vi "Read Sensors V.3.0.vi"(1 "Left Dart Motor":T1={"DeviceStatus"={"status"=FALSE, "code"=0, "source"=""}, "Type"=enum."PWM", "PWM"={"PWM Channel"=enum."Invalid", "DeadBand"={"Name"="", "maxPositivePwm"=0, "minPositivePwm"=0, "centerPwm"=0, "maxNegativePwm"=0, "minNegativePwm"=0, "angularRange"=0}}, "CAN"={"Device Number"=0, "SetOutput VI Ref"=variant(enum8{"Percent VBus", "Current", "Speed", "Position", "Voltage"} enum."Percent VBus"), "GetOutput VI Ref"=variant(refnum<k1> refnum), "Enable VI Ref"=variant(dbl 12.0), "Disable VI Ref"=variant(enum8{"Percent VBus", "Speed", "Position", "Slave", "Unchanged / Invalid", "Voltage Compensation", "Current", "Motion Profile"} enum."Percent VBus"), "Data"=variant}, "Invert"=FALSE, "DIO PWM"={"PWM \"Enable\" Channel"=enum."Invalid", "DIOChannel"=enum."Invalid", "PWM Rate"=0.0}}, 2 "Right Dart Motor":T1={"DeviceStatus"={"status"=FALSE, "code"=0, "source"=""}, "Type"=enum."PWM", "PWM"={"PWM Channel"=enum."Invalid", "DeadBand"={"Name"="", "maxPositivePwm"=0, "minPositivePwm"=0, "centerPwm"=0, "maxNegativePwm"=0, "minNegativePwm"=0, "angularRange"=0}}, "CAN"={"Device Number"=0, "SetOutput VI Ref"=variant(enum8{"Percent VBus", "Current", "Speed", "Position", "Voltage"} enum."Percent VBus"), "GetOutput VI Ref"=variant(refnum<k1> refnum), "Enable VI Ref"=variant(dbl 12.0), "Disable VI Ref"=variant(enum8{"Percent VBus", "Speed", "Position", "Slave", "Unchanged / Invalid", "Voltage Compensation", "Current", "Motion Profile"} enum."Percent VBus"), "Data"=variant}, "Invert"=FALSE, "DIO PWM"={"PWM \"Enable\" Channel"=enum."Invalid", "DIOChannel"=enum."Invalid", "PWM Rate"=0.0}}, 3 "Right Collector Intake Motor":T1={"DeviceStatus"={"status"=FALSE, "code"=0, "source"=""}, "Type"=enum."PWM", "PWM"={"PWM Channel"=enum."Invalid", "DeadBand"={"Name"="", "maxPositivePwm"=0, "minPositivePwm"=0, "centerPwm"=0, "maxNegativePwm"=0, "minNegativePwm"=0, "angularRange"=0}}, "CAN"={"Device Number"=0, "SetOutput VI Ref"=variant(enum8{"Percent VBus", "Current", "Speed", "Position", "Voltage"} enum."Percent VBus"), "GetOutput VI Ref"=variant(refnum<k1> refnum), "Enable VI Ref"=variant(dbl 12.0), "Disable VI Ref"=variant(enum8{"Percent VBus", "Speed", "Position", "Slave", "Unchanged / Invalid", "Voltage Compensation", "Current", "Motion Profile"} enum."Percent VBus"), "Data"=variant}, "Invert"=FALSE, "DIO PWM"={"PWM \"Enable\" Channel"=enum."Invalid", "DIOChannel"=enum."Invalid", "PWM Rate"=0.0}}, 4 "Right Pot.":T6, 5 "Left Collector Intake Motor":T1={"DeviceStatus"={"status"=FALSE, "code"=0, "source"=""}, "Type"=enum."PWM", "PWM"={"PWM Channel"=enum."Invalid", "DeadBand"={"Name"="", "maxPositivePwm"=0, "minPositivePwm"=0, "centerPwm"=0, "maxNegativePwm"=0, "minNegativePwm"=0, "angularRange"=0}}, "CAN"={"Device Number"=0, "SetOutput VI Ref"=variant(enum8{"Percent VBus", "Current", "Speed", "Position", "Voltage"} enum."Percent VBus"), "GetOutput VI Ref"=variant(refnum<k1> refnum), "Enable VI Ref"=variant(dbl 12.0), "Disable VI Ref"=variant(enum8{"Percent VBus", "Speed", "Position", "Slave", "Unchanged / Invalid", "Voltage Compensation", "Current", "Motion Profile"} enum."Percent VBus"), "Data"=variant}, "Invert"=FALSE, "DIO PWM"={"PWM \"Enable\" Channel"=enum."Invalid", "DIOChannel"=enum."Invalid", "PWM Rate"=0.0}}, 6 "Left Pot.":T6) -> ()   [LabVIEW 2017]
uses:
  <vilib>/Rock Robotics/WPI/Potentiometer/WPI_PotentiometerDevRef.ctl
  <vilib>/Rock Robotics/SystemInterfaces/AI/FPGA_AIChannel.ctl
  <vilib>/Rock Robotics/WPI/MotorControl/WPI_MotorControlDeviceRef.ctl
  <vilib>/Rock Robotics/WPI/MotorControl/WPI_MotorControlType.ctl
  <vilib>/Rock Robotics/SystemInterfaces/DIO/FPGA_DIOPWMChannel.ctl
  <vilib>/Rock Robotics/WPI/PWM/WPI_PWMDeadband.ctl
  <vilib>/Rock Robotics/SystemInterfaces/DIO/FPGA_DIOChannel.ctl
  Robot Global Data V.3.0.vi
  Public/Documents/Cross The Road Electronics/Phoenix-LabVIEW/Motor Controller/Get/CTRE_Phoenix_MotorController_GetOutputCurrent_Enhanced.vi
  Public/Documents/Cross The Road Electronics/Phoenix-LabVIEW/Motor Controller/Get/CTRE_Phoenix_MotorController_GetQuadratureData.vi
  <vilib>/Rock Robotics/WPI/Utilities/WPI_GetSetVariantRefNum.vi
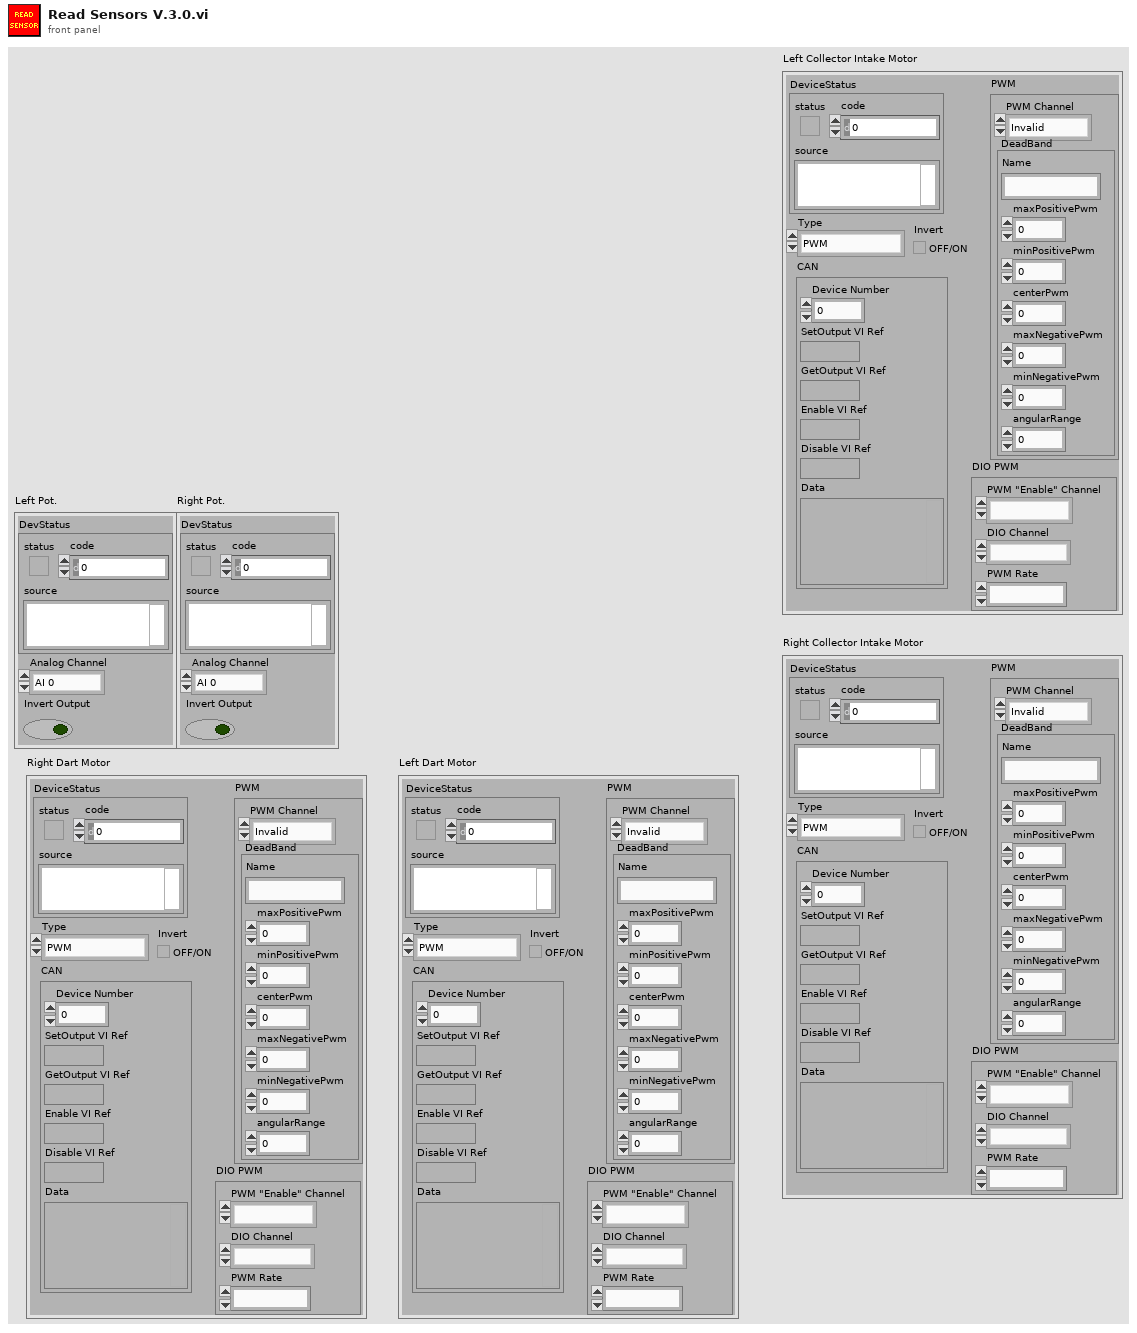
[diagram p1: front panel]
types:
  T1 = typedef "WPI_MotorControlDeviceRef.ctl" = cluster{"DeviceStatus":errorcluster, "Type":T2, "PWM":cluster{"PWM Channel":T3, "DeadBand":T4}, "CAN":cluster{"Device Number":u8, "SetOutput VI Ref":variant, "GetOutput VI Ref":variant, "Enable VI Ref":variant, "Disable VI Ref":variant, "Data":variant}, "Invert":bool, "DIO PWM":cluster{"PWM \"Enable\" Channel":T3, "DIOChannel":T5, "PWM Rate":dbl}}
  T2 = typedef "WPI_MotorControlType.ctl" = enum16{"PWM", "CAN", "DIO PWM"}
  T3 = typedef "FPGA_DIOPWMChannel.ctl" = enum8{"PWM 0", "PWM 1", "PWM 2", "PWM 3", "PWM 4", "PWM 5", "PWM 6", "PWM 7", "PWM 8", "PWM 9", "PWM MXP 0", "PWM MXP 1", "PWM MXP 2", "PWM MXP 3", "PWM MXP 4", "PWM MXP 5", "PWM MXP 6", "PWM MXP 7", "PWM MXP 8", "PWM MXP 9", "Invalid"}
  T4 = typedef "WPI_PWMDeadband.ctl" = cluster{"Name":string, "maxPositivePwm":i32, "minPositivePwm":i32, "centerPwm":i32, "maxNegativePwm":i32, "minNegativePwm":i32, "angularRange":u16}
  T5 = typedef "FPGA_DIOChannel.ctl" = enum8{"DIO 0", "DIO 1", "DIO 2", "DIO 3", "DIO 4", "DIO 5", "DIO 6", "DIO 7", "DIO 8", "DIO 9", "DIO MXP 0", "DIO MXP 1", "DIO MXP 2", "DIO MXP 3", "DIO MXP 4", "DIO MXP 5", "DIO MXP 6", "DIO MXP 7", "DIO MXP 8", "DIO MXP 9", "DIO MXP 10", "DIO MXP 11", "DIO MXP 12", "DIO MXP 13", "DIO MXP 14", "DIO MXP 15", "SPI Port CS1", "SPI Port CS2", "SPI Port CS3", "SPI Port MISO", "SPI Port MOSI", "Invalid"}
  T6 = typedef "WPI_PotentiometerDevRef.ctl" = cluster{"DevStatus":errorcluster, "Analog Channel":T7, "Invert Output":bool}
  T7 = typedef "FPGA_AIChannel.ctl" = enum8{"AI 0", "AI 1", "AI 2", "AI 3", "AI MXP 0", "AI MXP 1", "AI MXP 2", "AI MXP 3", "Invalid"}
  T8 = cluster{"Pot. Voltage":dbl[], "Corresponding Inches":dbl[]}
  T9 = typedef "WPI_RobotDriveDevRef.ctl" = cluster{"DevStatus":errorcluster, "Motors[]":T1[], "Square Inputs":bool, "Max Output":dbl}
  T10 = typedef "WPI_GyroDevRef.ctl" = cluster{"DevStatus":errorcluster, "Analog Channel":T7, "Gain (VoltsPerDegree/Second)":dbl, "Gyro Type":enum16{"Analog", "XRS450"}, "Handle":i32, "SPI Bus":T11, "Device Found":bool, "Sample Rate":dbl, "Calibrate On Open":bool, "Offset":dbl}
  T11 = typedef "spi_bus.ctl" = enum16{"SPI On-Board, CS0", "SPI On-Board, CS1", "SPI On-Board, CS2", "SPI On-Board, CS3", "SPI MXP", "Invalid"}
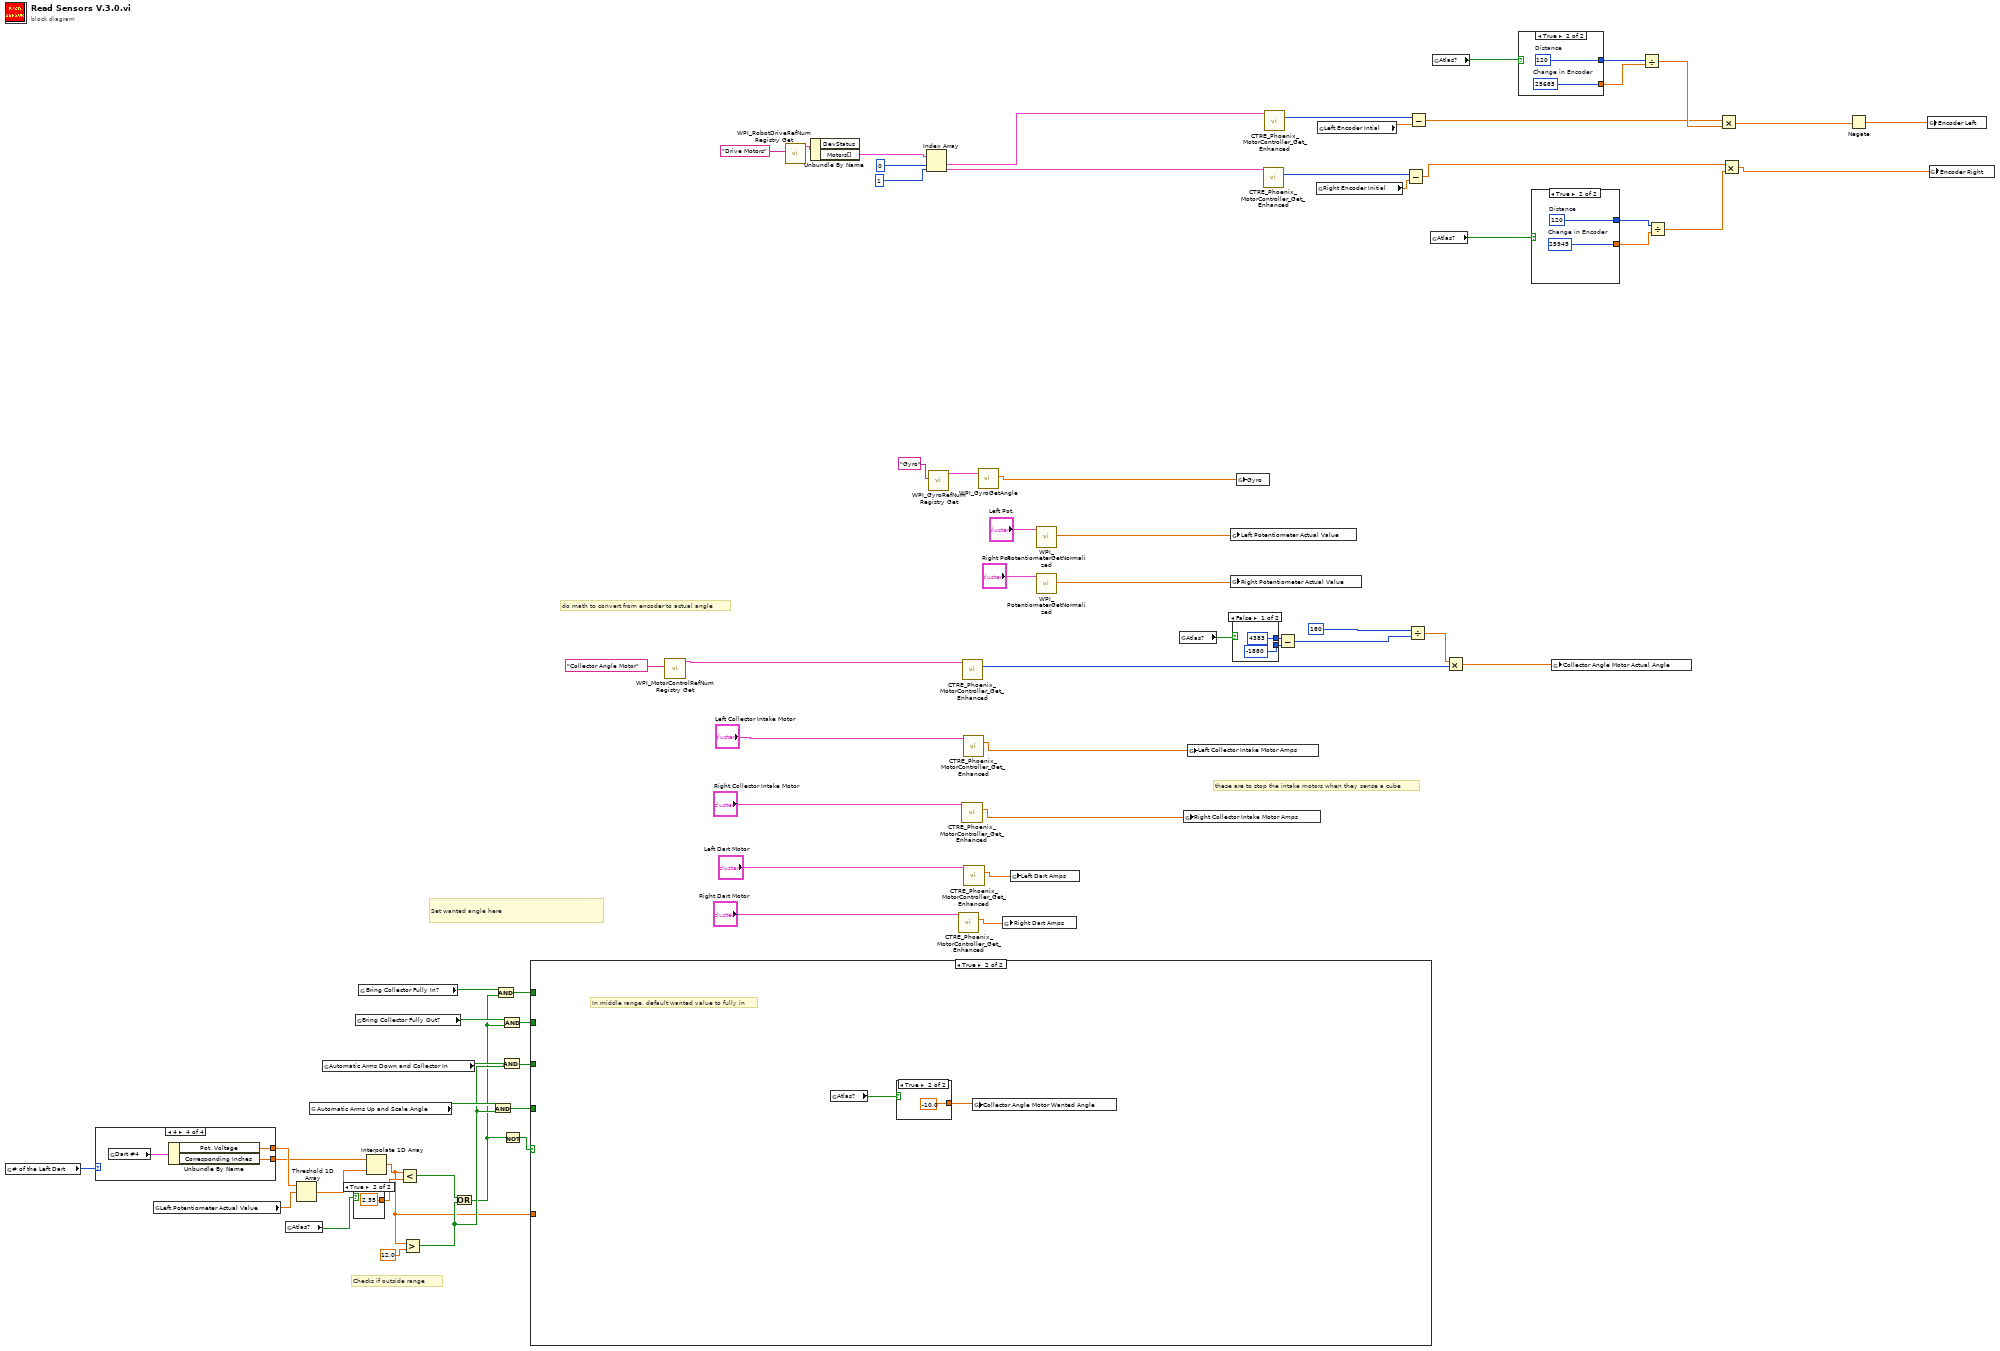
[diagram p0: block diagram]
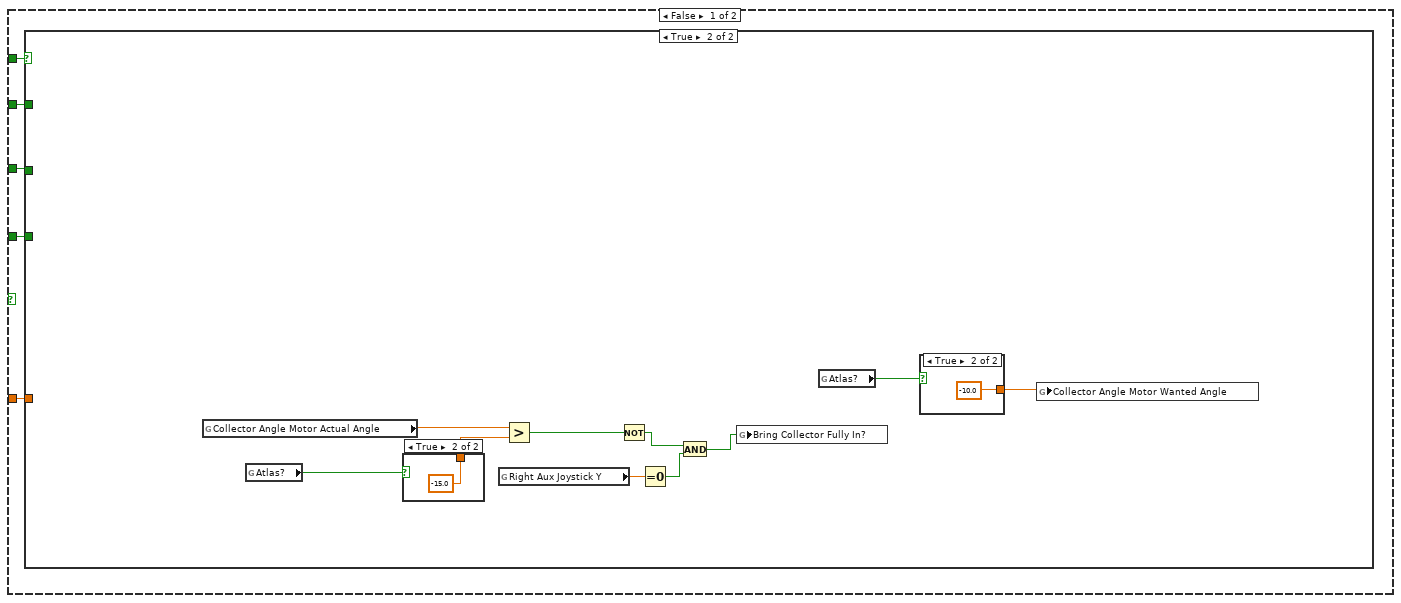
[diagram p2: hidden frame]
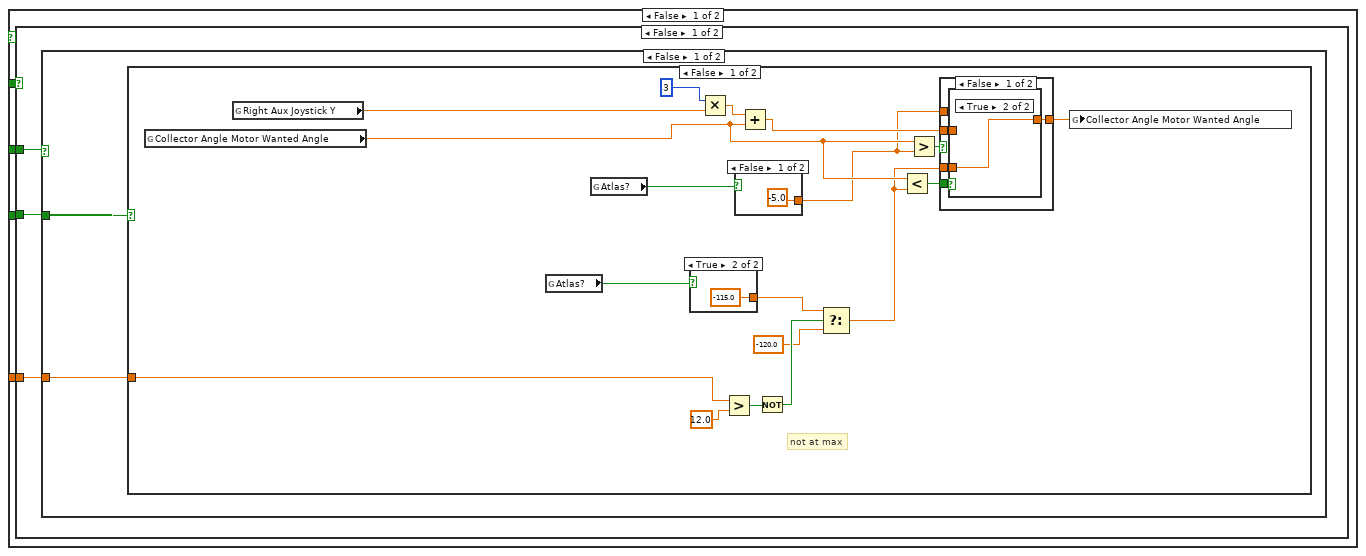
[diagram p3: hidden frame]
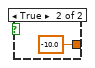
[diagram p4: hidden frame]
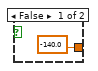
[diagram p5: hidden frame]
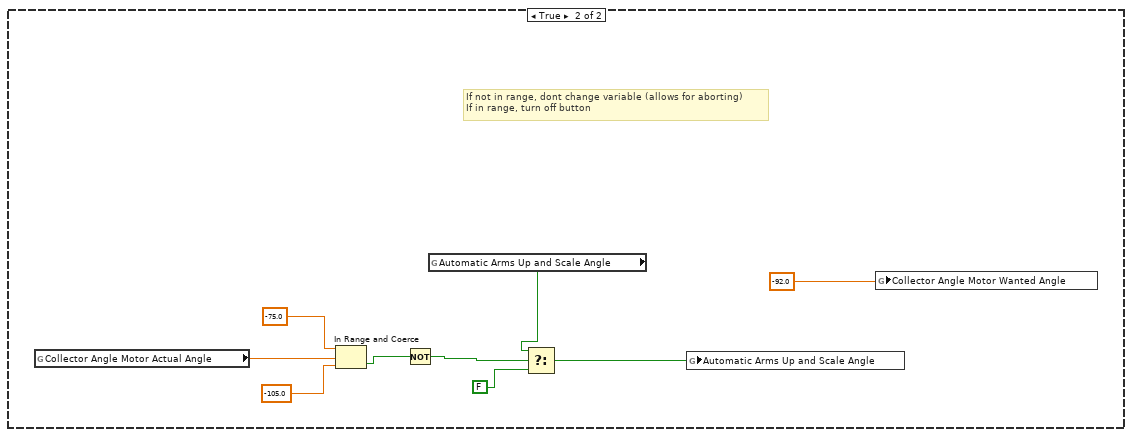
[diagram p8: hidden frame]
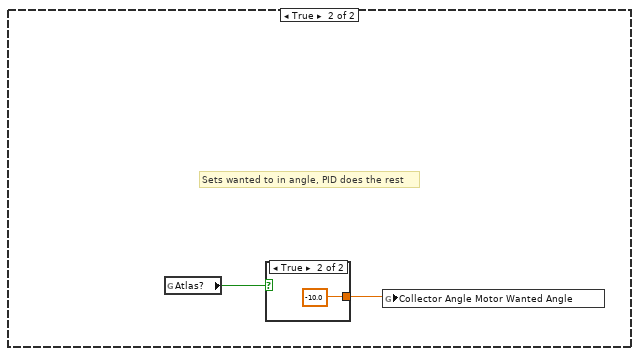
[diagram p9: hidden frame]
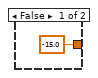
[diagram p10: hidden frame]
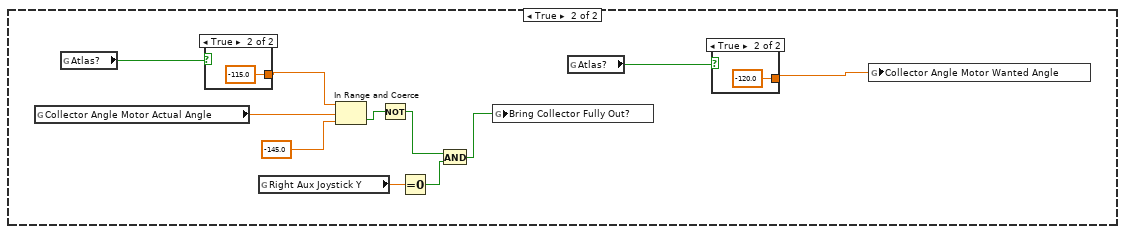
[diagram p11: hidden frame]
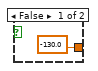
[diagram p12: hidden frame]
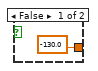
[diagram p13: hidden frame]
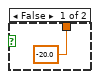
[diagram p14: hidden frame]
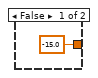
[diagram p15: hidden frame]
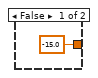
[diagram p16: hidden frame]
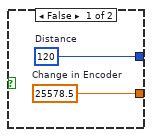
[diagram p17: hidden frame]
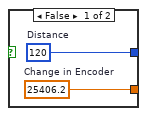
[diagram p18: hidden frame]
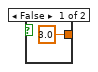
[diagram p19: hidden frame]
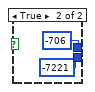
[diagram p20: hidden frame]
diagram:
  # "Checks if outside range"
  # "Set wanted angle here"
  # "these are to stop the intake motors when they sense a cube"
  # "do math to convert from encoder to actual angle"
  n1 = global read "Robot Global Data V.3.0.vi" "# of the Left Dart"() -> (w29:i32)
  n2 = case shown="4" w29 {
    tunnel: [w72 w75 w78 w81] -> w31
    tunnel: [w71 w74 w77 w80] -> w30
    frame 1, Default {
      n3 = global read "Robot Global Data V.3.0.vi" "Dart #1"() -> (w73:T8)
      n4 = Unbundle By Name(w73) -> ("Pot. Voltage"=w72:dbl[], "Corresponding Inches"=w71:dbl[])
    }
    frame 2 {
      n5 = global read "Robot Global Data V.3.0.vi" "Dart #2"() -> (w76:T8)
      n6 = Unbundle By Name(w76) -> ("Pot. Voltage"=w75:dbl[], "Corresponding Inches"=w74:dbl[])
    }
    frame 3 {
      n7 = global read "Robot Global Data V.3.0.vi" "Dart #3"() -> (w79:T8)
      n8 = Unbundle By Name(w79) -> ("Pot. Voltage"=w78:dbl[], "Corresponding Inches"=w77:dbl[])
    }
    frame 4 {
      n9 = global read "Robot Global Data V.3.0.vi" "Dart #4"() -> (w82:T8)
      n10 = Unbundle By Name(w82) -> ("Pot. Voltage"=w81:dbl[], "Corresponding Inches"=w80:dbl[])
    }
  }
  n11 = global read "Robot Global Data V.3.0.vi" "Left Potentiometer Actual Value"() -> (w32:dbl)
  n12 = global read "Robot Global Data V.3.0.vi" "Atlas?"() -> (w14:bool)
  n13 = Threshold 1D Array(2:w32, 3:w31) -> (0:w33:dbl)  [unwired: 1 in]
  n14 = global read "Robot Global Data V.3.0.vi" "Automatic Arms Up and Scale Angle"() -> (w16:bool)
  n15 = global read "Robot Global Data V.3.0.vi" "Automatic Arms Down and Collector In"() -> (w8:bool)
  n16 = case shown="True" w14 {
    tunnel: [3.0 ("y") 2.35 ("y")] -> w28
    frame False {
    }
    frame True {
    }
  }
  n17 = global read "Robot Global Data V.3.0.vi" "Bring Collector Fully Out?"() -> (w24:bool)
  n18 = global read "Robot Global Data V.3.0.vi" "Bring Collector Fully In?"() -> (w25:bool)
  n19 = Interpolate 1D Array(1:w33, 2:w30) -> (0:w3:dbl)
  n20 = Less?(x=w3, y=w28) -> (x < y?=w26:bool)
  n21 = Greater?(x=w3, y=12.0) -> (0:w6:bool)
  n22 = Or(x=w26, y=w6) -> (x .or. y?=w1:bool)
  n23 = And(x=w16, y=w6) -> (x .and. y?=w11:bool)
  n24 = And(x=w25, y=w1) -> (x .and. y?=w13:bool)
  n25 = And(x=w8, y=w6) -> (x .and. y?=w7:bool)
  n26 = And(x=w24, y=w1) -> (x .and. y?=w12:bool)
  n27 = Not(x=w1) -> (.not. x?=w2:bool)
  n28 = case shown="True" w2 {
    tunnel: w13 -> [w89 _]
    tunnel: w12 -> [w88 _]
    tunnel: w11 -> [w87 _]
    tunnel: w7 -> [w86 _]
    tunnel: w3 -> [w85 _]
    frame False {
      n29 = case shown="True" w89 {
        tunnel: w88 -> [w93 _]
        tunnel: w86 -> [w92 _]
        tunnel: w87 -> [w91 _]
        tunnel: w85 -> [w90 _]
        frame False {
          n30 = case shown="False" w93 {
            tunnel: w92 -> [w96 _]
            tunnel: w91 -> [w95 _]
            tunnel: w90 -> [w94 _]
            frame False {
              n31 = case shown="False" w96 {
                tunnel: w95 -> [w98 _]
                tunnel: w94 -> [w97 _]
                frame False {
                  n32 = case shown="False" w98 {
                    tunnel: w97 -> [w101 _]
                    frame False {
                      # "not at max"
                      n33 = global read "Robot Global Data V.3.0.vi" "Collector Angle Motor Wanted Angle"() -> (w110:dbl)
                      n34 = global read "Robot Global Data V.3.0.vi" "Right Aux Joystick Y"() -> (w116:dbl)
                      n35 = global read "Robot Global Data V.3.0.vi" "Atlas?"() -> (w102:bool)
                      n36 = global read "Robot Global Data V.3.0.vi" "Atlas?"() -> (w100:bool)
                      n37 = case shown="True" w102 {
                        tunnel: [-140.0 ("t") -115.0 ("t")] -> w105
                        frame False {
                        }
                        frame True {
                        }
                      }
                      n38 = Multiply(x=3, y=w116) -> (x*y=w115:dbl)
                      n39 = Greater?(x=w101, y=12.0) -> (0:w107:bool)
                      n40 = case shown="False" w100 {
                        tunnel: [-5.0 ("t") -10.0 ("t")] -> w99
                        frame False {
                        }
                        frame True {
                        }
                      }
                      n41 = Add(x=w115, y=w110) -> (x+y=w113:dbl)
                      n42 = Not(x=w107) -> (.not. x?=w106:bool)
                      n43 = Select(t=w105, s=w106, f=-120.0) -> (s? t:f=w103:dbl)
                      n44 = Less?(x=w110, y=w103) -> (x < y?=w109:bool)
                      n45 = Greater?(x=w110, y=w99) -> (0:w112:bool)
                      n46 = case shown="False" w112 {
                        tunnel: w99 -> [_ w127]
                        tunnel: w113 -> [w121 _]
                        tunnel: [w123 w127] -> w111
                        tunnel: w109 -> [w124 _]
                        tunnel: w103 -> [w122 _]
                        frame False {
                          n47 = case shown="True" w124 {
                            tunnel: [w125 w126] -> w123
                            tunnel: w122 -> [_ w126]
                            tunnel: w121 -> [w125 _]
                            frame False {
                            }
                            frame True {
                            }
                          }
                        }
                        frame True {
                        }
                      }
                      n48 = global write "Robot Global Data V.3.0.vi" "Collector Angle Motor Wanted Angle"(w111) -> ()
                    }
                    frame True {
                      # "If not in range, dont change variable (allows for aborting)\nIf in range, turn off button"
                      n49 = global read "Robot Global Data V.3.0.vi" "Collector Angle Motor Actual Angle"() -> (w134:dbl)
                      n50 = In Range and Coerce(upper limit=-75.0, x=w134, lower limit=-105.0) -> (In Range?=w135:bool)  [unwired: 1 out]
                      n51 = Not(x=w135) -> (.not. x?=w131:bool)
                      n52 = global read "Robot Global Data V.3.0.vi" "Automatic Arms Up and Scale Angle"() -> (w129:bool)
                      n53 = Select(t=w129, s=w131, f=FALSE) -> (s? t:f=w130:bool)
                      n54 = global write "Robot Global Data V.3.0.vi" "Automatic Arms Up and Scale Angle"(w130) -> ()
                      n55 = global write "Robot Global Data V.3.0.vi" "Collector Angle Motor Wanted Angle"(-92.0) -> ()
                    }
                  }
                }
                frame True {
                  # "Sets wanted to in angle, PID does the rest"
                  n56 = global read "Robot Global Data V.3.0.vi" "Atlas?"() -> (w137:bool)
                  n57 = case shown="True" w137 {
                    tunnel: [-15.0 -10.0] -> w138
                    frame False {
                    }
                    frame True {
                    }
                  }
                  n58 = global write "Robot Global Data V.3.0.vi" "Collector Angle Motor Wanted Angle"(w138) -> ()
                }
              }
            }
            frame True {
              n59 = global read "Robot Global Data V.3.0.vi" "Collector Angle Motor Actual Angle"() -> (w150:dbl)
              n60 = global read "Robot Global Data V.3.0.vi" "Atlas?"() -> (w142:bool)
              n61 = case shown="True" w142 {
                tunnel: [-130.0 ("t") -115.0 ("t")] -> w141
                frame False {
                }
                frame True {
                }
              }
              n62 = global read "Robot Global Data V.3.0.vi" "Right Aux Joystick Y"() -> (w148:dbl)
              n63 = In Range and Coerce(upper limit=w141, x=w150, lower limit=-145.0) -> (In Range?=w151:bool)  [unwired: 1 out]
              n64 = Not(x=w151) -> (.not. x?=w146:bool)
              n65 = Equal To 0?(x=w148) -> (x = 0?=w147:bool)
              n66 = And(x=w146, y=w147) -> (x .and. y?=w145:bool)
              n67 = global write "Robot Global Data V.3.0.vi" "Bring Collector Fully Out?"(w145) -> ()
              n68 = global read "Robot Global Data V.3.0.vi" "Atlas?"() -> (w144:bool)
              n69 = case shown="True" w144 {
                tunnel: [-130.0 ("t") -120.0 ("t")] -> w143
                frame False {
                }
                frame True {
                }
              }
              n70 = global write "Robot Global Data V.3.0.vi" "Collector Angle Motor Wanted Angle"(w143) -> ()
            }
          }
        }
        frame True {
          n71 = global read "Robot Global Data V.3.0.vi" "Collector Angle Motor Actual Angle"() -> (w163:dbl)
          n72 = global read "Robot Global Data V.3.0.vi" "Atlas?"() -> (w161:bool)
          n73 = case shown="True" w161 {
            tunnel: [-20.0 -15.0] -> w162
            frame False {
            }
            frame True {
            }
          }
          n74 = global read "Robot Global Data V.3.0.vi" "Right Aux Joystick Y"() -> (w159:dbl)
          n75 = Greater?(x=w163, y=w162) -> (0:w164:bool)
          n76 = Not(x=w164) -> (.not. x?=w157:bool)
          n77 = Equal To 0?(x=w159) -> (x = 0?=w158:bool)
          n78 = And(x=w157, y=w158) -> (x .and. y?=w156:bool)
          n79 = global write "Robot Global Data V.3.0.vi" "Bring Collector Fully In?"(w156) -> ()
          n80 = global read "Robot Global Data V.3.0.vi" "Atlas?"() -> (w160:bool)
          n81 = case shown="True" w160 {
            tunnel: [-15.0 -10.0] -> w165
            frame False {
            }
            frame True {
            }
          }
          n82 = global write "Robot Global Data V.3.0.vi" "Collector Angle Motor Wanted Angle"(w165) -> ()
        }
      }
    }
    frame True {
      # "In middle range, default wanted value to fully in"
      n83 = global read "Robot Global Data V.3.0.vi" "Atlas?"() -> (w170:bool)
      n84 = case shown="True" w170 {
        tunnel: [-15.0 -10.0] -> w171
        frame False {
        }
        frame True {
        }
      }
      n85 = global write "Robot Global Data V.3.0.vi" "Collector Angle Motor Wanted Angle"(w171) -> ()
    }
  }
  n86 = call <vilib>:"WPI_MotorControlRefNum Registry Get.vi"("refnum name"="Collector Angle Motor") -> ("MotorControlDevRef"=w64:T1)  [unwired: 9 in, 1 out]
  n87 = call <vilib>:"WPI_RobotDriveRefNum Registry Get.vi"("refnum name"="Drive Motors") -> ("RobotDriveDevRef"=w62:T9)  [unwired: 9 in, 1 out]
  n88 = Unbundle By Name(w62) -> ("Motors[]"=w60:T1[])  [unwired: 1 out]
  n89 = Index Array(array=w60, index #1=0, index #2=1) -> (element #1=w57:T1, element #2=w56:T1)
  n90 = call <vilib>:"WPI_GyroRefNum Registry Get.vi"("refnum name"="Gyro") -> ("GyroDevRef"=w41:T10)  [unwired: 9 in, 1 out]
  n91 = call-poly "CTRE_Phoenix_MotorController_Get_Enhanced.vi"("PhoenixMotorControlDevRef"="Right Dart Motor") -> ("Output Current"=w48:dbl)  [unwired: 12 in, 2 out]
  n92 = call-poly "CTRE_Phoenix_MotorController_Get_Enhanced.vi"("PhoenixMotorControlDevRef"="Right Collector Intake Motor") -> ("Output Current"=w51:dbl)  [unwired: 12 in, 2 out]
  n93 = call-poly "CTRE_Phoenix_MotorController_Get_Enhanced.vi"("PhoenixMotorControlDevRef"=w64) -> ("Quadrature Position"=w53:i32)  [unwired: 11 in, 3 out]
  n94 = call-poly "CTRE_Phoenix_MotorController_Get_Enhanced.vi"("PhoenixMotorControlDevRef"="Left Collector Intake Motor") -> ("Output Current"=w52:dbl)  [unwired: 12 in, 2 out]
  n95 = call-poly "CTRE_Phoenix_MotorController_Get_Enhanced.vi"("PhoenixMotorControlDevRef"="Left Dart Motor") -> ("Output Current"=w49:dbl)  [unwired: 12 in, 2 out]
  n96 = call <vilib>:"WPI_GyroGetAngle.vi"("GyroDevRef"=w41) -> ("Angle"=w39:dbl)  [unwired: 6 in, 4 out]
  n97 = global write "Robot Global Data V.3.0.vi" "Right Dart Amps"(w48) -> ()
  n98 = global write "Robot Global Data V.3.0.vi" "Left Dart Amps"(w49) -> ()
  n99 = call <vilib>:"WPI_PotentiometerGetNormalized.vi"("PotDevRef"="Left Pot.") -> ("Normalized Value"=w70:dbl)  [unwired: 8 in, 2 out]
  n100 = call <vilib>:"WPI_PotentiometerGetNormalized.vi"("PotDevRef"="Right Pot.") -> ("Normalized Value"=w68:dbl)  [unwired: 8 in, 2 out]
  n101 = global read "Robot Global Data V.3.0.vi" "Atlas?"() -> (w15:bool)
  n102 = global write "Robot Global Data V.3.0.vi" "Right Collector Intake Motor Amps"(w51) -> ()
  n103 = global write "Robot Global Data V.3.0.vi" "Left Collector Intake Motor Amps"(w52) -> ()
  n104 = global write "Robot Global Data V.3.0.vi" "Left Potentiometer Actual Value"(w70) -> ()
  n105 = global write "Robot Global Data V.3.0.vi" "Right Potentiometer Actual Value"(w68) -> ()
  n106 = case shown="False" w15 {
    tunnel: [4383 -706] -> w43
    tunnel: [-1880 -7221] -> w42
    frame False {
    }
    frame True {
    }
  }
  n107 = global write "Robot Global Data V.3.0.vi" "Gyro"(w39) -> ()
  n108 = call-poly "CTRE_Phoenix_MotorController_Get_Enhanced.vi"("PhoenixMotorControlDevRef"=w56) -> ("Quadrature Position"=w20:i32)  [unwired: 11 in, 3 out]
  n109 = call-poly "CTRE_Phoenix_MotorController_Get_Enhanced.vi"("PhoenixMotorControlDevRef"=w57) -> ("Quadrature Position"=w23:i32)  [unwired: 11 in, 3 out]
  n110 = Subtract(x=w43, y=w42) -> (x-y=w44:i32)
  n111 = global read "Robot Global Data V.3.0.vi" "Right Encoder Initial"() -> (w19:dbl)
  n112 = global read "Robot Global Data V.3.0.vi" "Left Encoder Intial"() -> (w22:dbl)
  n113 = Subtract(x=w20, y=w19) -> (x-y=w17:dbl)
  n114 = Divide(x=180, y=w44) -> (x/y=w45:dbl)
  n115 = Subtract(x=w23, y=w22) -> (x-y=w21:dbl)
  n116 = global read "Robot Global Data V.3.0.vi" "Atlas?"() -> (w10:bool)
  n117 = global read "Robot Global Data V.3.0.vi" "Atlas?"() -> (w9:bool)
  n118 = Multiply(x=w45, y=w53) -> (x*y=w54:dbl)
  n119 = case shown="True" w9 {
    tunnel: [w179 w181] -> w38
    tunnel: [w178 w180] -> w37
    frame False {
      w178 = 25406.2  # Change in Encoder
      w179 = 120  # Distance
    }
    frame True {
      w180 = 25685  # Change in Encoder
      w181 = 120  # Distance
    }
  }
  n120 = case shown="True" w10 {
    tunnel: [w182 w185] -> w35
    tunnel: [w183 w184] -> w34
    frame False {
      w182 = 25578.5  # Change in Encoder
      w183 = 120  # Distance
    }
    frame True {
      w185 = 25945  # Change in Encoder
      w184 = 120  # Distance
    }
  }
  n121 = global write "Robot Global Data V.3.0.vi" "Collector Angle Motor Actual Angle"(w54) -> ()
  n122 = Divide(x=w38, y=w37) -> (x/y=w36:dbl)
  n123 = Divide(x=w34, y=w35) -> (x/y=w18:dbl)
  n124 = Multiply(x=w21, y=w36) -> (x*y=w5:dbl)
  n125 = Multiply(x=w17, y=w18) -> (x*y=w55:dbl)
  n126 = Negate(x=w5) -> (-x=w4:dbl)
  n127 = global write "Robot Global Data V.3.0.vi" "Encoder Left"(w4) -> ()
  n128 = global write "Robot Global Data V.3.0.vi" "Encoder Right"(w55) -> ()
